vi "Teleop.vi"(10 "Match Info":T1={"Autonomous Elapsed Seconds"=0.0, "TeleOp Elapsed Seconds"=72.473, "Disabled Elapsed Seconds"=26.679, "Visited Autonomous"=FALSE, "Visited TeleOp"=TRUE, "Visited Disabled"=TRUE, "Autonomous Settings"={"Autonomous Style"=enum."Independent", "VI Refnum"=refnum}}, 11 "Call Context":T2=enum."Stop") -> ()   [LabVIEW 2014]
doc: "This VI is called for each TeleOp packet received from the DS where the robot is not disabled. It is often used to read from the joysticks and update I/O or to update setpoints for timed control loops. It should complete and return within 20 milliseconds or it may miss DS packets."
uses:
  Robot Global Data.vi
  <vilib>/Rock Robotics/WPI/SafetyOutput/WPI_SafetyOutputConfigMenu.ctl
  <vilib>/Rock Robotics/WPI/Solenoid/Deprecated/WPI_SolenoidSetBool.vi
  <vilib>/Rock Robotics/WPI/DriverStation/WPI_DriverStationMatch Info.ctl
  <vilib>/Rock Robotics/WPI/DriverStation/WPI_DriverStationDerivedRobotMode.ctl
panel:
  in  "Feed_Forwards_Speed":dbl=0.75 step=0.05
  in  "Feed_Backwards_Speed":dbl=-0.5 step=0.05
  in  "Override_Feed_Value":dbl=1.0
  in  "Override_Feed_Enable":bool
  in  "Mantis_Arm_Control_Rate":dbl=20.0
  out "Delta_Time":dbl=0.023
  in  "Triger_Fire_Threshold":dbl=0.6 format="%#_13g"
  in  "Mantis_Arms_Full_Forward_Position":dbl=69.0
  in  "Mantis_Arms_Full_Back_Position":dbl=100.0
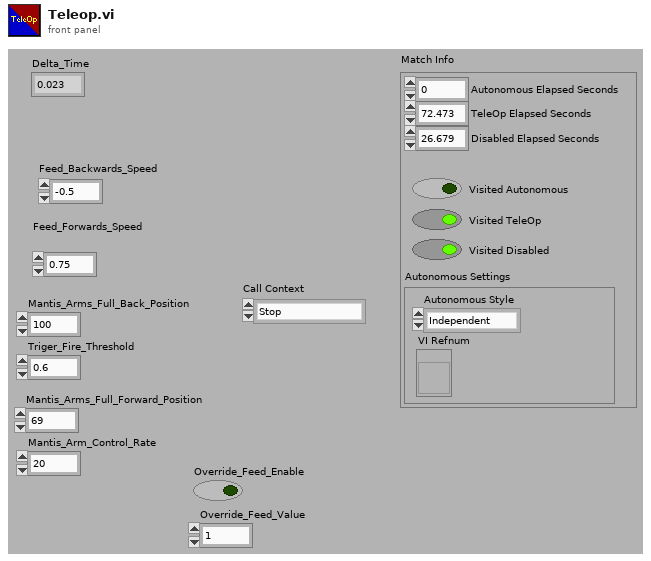
[diagram p1: front panel]
types:
  T1 = typedef "WPI_DriverStationMatch Info.ctl" = cluster{"Autonomous Elapsed Seconds":dbl, "TeleOp Elapsed Seconds":dbl, "Disabled Elapsed Seconds":dbl, "Visited Autonomous":bool, "Visited TeleOp":bool, "Visited Disabled":bool, "Autonomous Settings":cluster{"Autonomous Style":enum16{"Iterative", "Independent"}, "VI Refnum":refnum<vi>}}
  T2 = typedef "WPI_DriverStationDerivedRobotMode.ctl" = enum16{"Init", "Execute", "Stop"}
  T3 = typedef "WPI_SafetyOutputConfigMenu.ctl" = enum16{"Enable", "Disable"}
  T4 = typedef "WPI_RobotDriveDevRef.ctl" = cluster{"DevStatus":errorcluster, "Motors[]":T5[], "Square Inputs":bool, "Max Output":dbl}
  T5 = typedef "WPI_MotorControlDeviceRef.ctl" = cluster{"DeviceStatus":errorcluster, "Type":enum16{"PWM", "CAN"}, "PWM":cluster{"Digital Module":T6, "PWM Channel":T7, "DeadBand":T8}, "CAN":cluster{"Device Number":u8, "Control Mode":T9, "Semaphore":T10, "Max Vout":dbl}, "Invert":bool, "TransformRef":T11, "InvTransformRef":T11}
  T6 = typedef "FPGA_TypedefDigitalModule.ctl" = enum16{"Digital Module 1", "Digital Module 2"}
  T7 = typedef "FPGA_DIOPWMChannel.ctl" = enum8{"PWM 1", "PWM 2", "PWM 3", "PWM 4", "PWM 5", "PWM 6", "PWM 7", "PWM 8", "PWM 9", "PWM 10", "Invalid"}
  T8 = typedef "WPI_PWMDeadband.ctl" = cluster{"Name":string, "maxPositivePwm":i32, "minPositivePwm":i32, "centerPwm":i32, "maxNegativePwm":i32, "minNegativePwm":i32, "angularRange":u16}
  T9 = typedef "WPI_CANJaguar_ControlMode.ctl" = enum8{"Percent VBus", "Current", "Speed", "Position", "Voltage"}
  T10 = typedef "Semaphore RefNum" = refnum<k1>
  T11 = typedef "WPI_PWMTransform_ConPane.ctl" = refnum<vi>
  T12 = typedef "WPI_JoystickDevRef.ctl" = cluster{"Device":T13}
  T13 = typedef "WPI_JoystickDeviceEnum.ctl" = enum16{"USB 0", "USB 1", "USB 2", "USB 3", "USB 4", "USB 5"}
  T14 = cluster{"Button 1":bool, "Button 2":bool, "Button 3":bool, "Button 4":bool, "Button 5":bool, "Button 6":bool, "Button 7":bool, "Button 8":bool, "Button 9":bool, "Button 10":bool, "Button 11":bool, "Button 12":bool}
  T15 = cluster{"axis 1 (x)":dbl, "axis 2 (y)":dbl, "axis 3 (throttle)":dbl, "axis 4":dbl, "axis 5":dbl, "axis 6":dbl}
  T16 = typedef "WPI_SolenoidDevRef.ctl" = cluster{"DevStatus":errorcluster, "Solenoid Module":T17, "Forward Solenoid Channel":T18, "Reverse Solenoid Channel":T18}
  T17 = typedef "FPGA_TypedefSolenoidModule.ctl" = enum16{"Solenoid Module 1", "Solenoid Module 2"}
  T18 = typedef "WPI_SolenoidChannel.ctl" = enum8{"Solenoid 1", "Solenoid 2", "Solenoid 3", "Solenoid 4", "Solenoid 5", "Solenoid 6", "Solenoid 7", "Solenoid 8", "Invalid"}
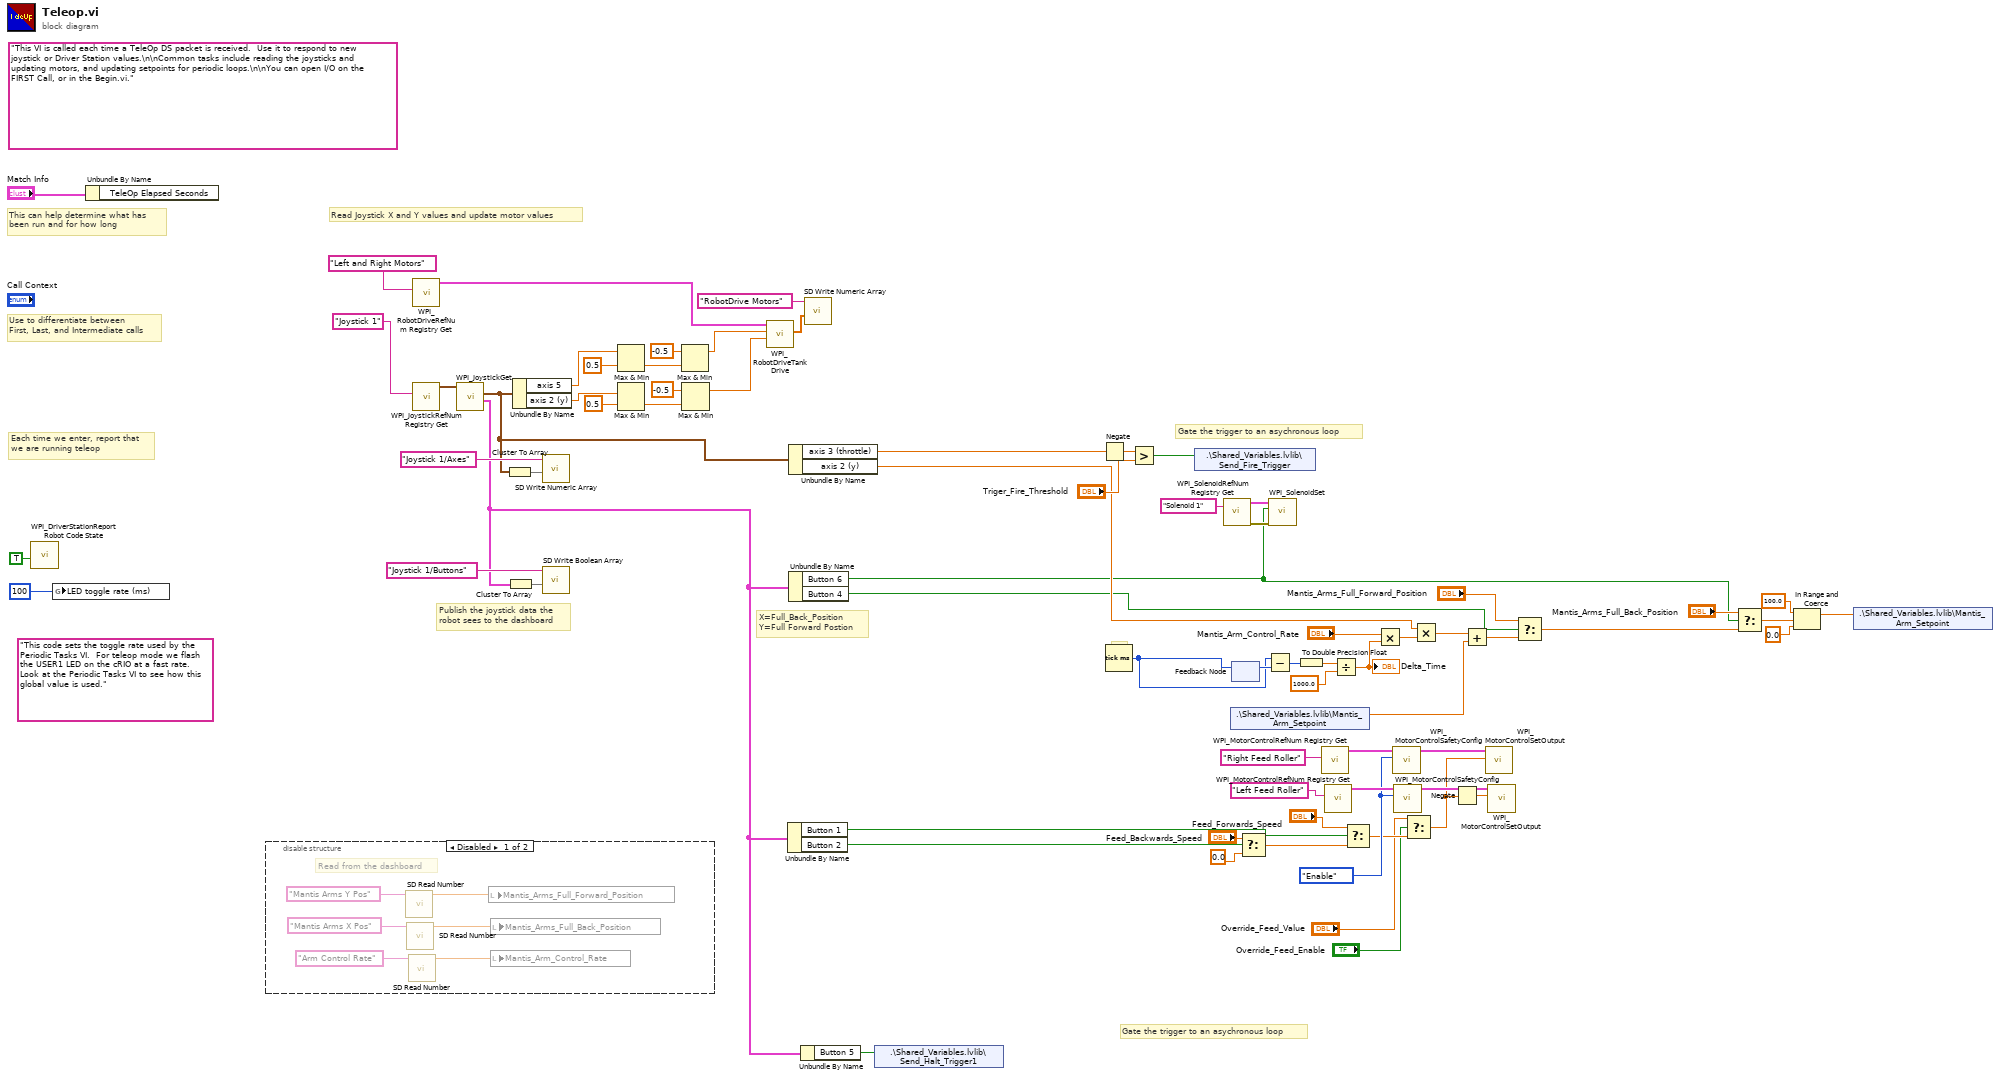
[diagram p0: block diagram]
diagram:
  w31 = WPI_SafetyOutputConfigMenu."Enable" ("mode")
  (unwired) "This code sets the toggle rate used by the Periodic Tasks VI.  For teleop mode we flash the USER1 LED on the cRIO at a fast rate.  Look at the Periodic Tasks VI to see how this global value is used."
  (unwired) "This VI is called each time a TeleOp DS packet is received.  Use it to respond to new joystick or Driver Station values.\n\nCommon tasks include reading the joysticks and updating motors, and updating setpoints for periodic loops.\n\nYou can open I/O on the FIRST Call, or in the Begin.vi."
  # "Gate the trigger to an asychronous loop"
  # "Gate the trigger to an asychronous loop"
  # "dT"
  # "X=Full_Back_Position\nY=Full Forward Postion"
  # "Publish the joystick data the\nrobot sees to the dashboard"
  # "Each time we enter, report that\nwe are running teleop"
  # "Use to differentiate between\nFirst, Last, and Intermediate calls"
  # "This can help determine what has\nbeen run and for how long"
  # "Read Joystick X and Y values and update motor values"
  n1 = call <vilib>:"WPI_DriverStationReport Robot Code State.vi"("TeleOp"=TRUE ("Autonomous")) -> ()  [unwired: 10 in, 1 out]
  n2 = global write "Robot Global Data.vi" "LED toggle rate (ms)"(u32 100 ("LED ms toggle rate")) -> ()
  n3 = Unbundle By Name("Match Info") -> ()  [unwired: 1 out]
  n4 = disable-structure shown="Disabled" {
    frame Disabled {
      # "Read from the dashboard"
      n5 = call <vilib>:"SD Read Number.vi"("Name"="Mantis Arms Y Pos" ("refnum name")) -> ("Numeric"=w74:dbl)  [unwired: 8 in, 2 out]
      n6 = call <vilib>:"SD Read Number.vi"("Name"="Mantis Arms X Pos" ("refnum name")) -> ("Numeric"=w76:dbl)  [unwired: 8 in, 2 out]
      n7 = call <vilib>:"SD Read Number.vi"("Name"="Arm Control Rate" ("refnum name")) -> ("Numeric"=w77:dbl)  [unwired: 8 in, 2 out]
      n8 = local write "Mantis_Arms_Full_Forward_Position"(w74) -> ()
      n9 = local write "Mantis_Arms_Full_Back_Position"(w76) -> ()
      n10 = local write "Mantis_Arm_Control_Rate"(w77) -> ()
    }
    frame Enabled {
    }
  }
  n11 = call <vilib>:"WPI_RobotDriveRefNum Registry Get.vi"("refnum name"="Left and Right Motors") -> ("RobotDriveDevRef"=w62:T4)  [unwired: 1 in, 9 out]
  n12 = call <vilib>:"WPI_JoystickRefNum Registry Get.vi"("refnum name"="Joystick 1") -> ("JoystickDevRef"=w69:T12)  [unwired: 1 in, 9 out]
  n13 = call <vilib>:"WPI_JoystickGet.vi"("JoystickDevRef"=w69) -> ("Buttons"=w12:T14, "Axes"=w11:T15)  [unwired: 1 in, 4 out]
  n14 = Cluster To Array(cluster=w11) -> (array=w64:dbl[])
  n15 = Cluster To Array(cluster=w12) -> (array=w66:bool[])
  n16 = Unbundle By Name(w11) -> ("axis 5"=w10:dbl, "axis 2 (y)"=w9:dbl)
  n17 = call <vilib>:"SD Write Numeric Array.vi"("Numeric Array"=w64, "Name"="Joystick 1/Axes") -> ()  [unwired: 8 in, 2 out]
  n18 = call <vilib>:"SD Write Boolean Array.vi"("Boolean Array"=w66, "Name"="Joystick 1/Buttons") -> ()  [unwired: 8 in, 2 out]
  n19 = Max & Min(x=w10, y=0.5) -> (min(x,y)=w6:dbl)  [unwired: 1 out]
  n20 = Max & Min(x=w9, y=0.5) -> (min(x,y)=w5:dbl)  [unwired: 1 out]
  n21 = Max & Min(x=-0.5, y=w6) -> (max(x,y)=w2:dbl)  [unwired: 1 out]
  n22 = Max & Min(x=-0.5, y=w5) -> (max(x,y)=w1:dbl)  [unwired: 1 out]
  n23 = call <vilib>:"WPI_RobotDriveTankDrive.vi"("Right axis value"=w1, "Left axis value"=w2, "RobotDriveDevRef"=w62) -> ("Motor Values"=w60:dbl[])  [unwired: 6 in, 2 out]
  n24 = Unbundle By Name(w12) -> ("Button 1"=w58:bool, "Button 2"=w57:bool)
  n25 = Unbundle By Name(w11) -> ("axis 3 (throttle)"=w55:dbl, "axis 2 (y)"=w43:dbl)
  n26 = Unbundle By Name(w12) -> ("Button 6"=w13:bool, "Button 4"=w14:bool)
  n27 = Unbundle By Name(w12) -> ("Button 5"=w20:bool)
  n28 = call <vilib>:"SD Write Numeric Array.vi"("Numeric Array"=w60, "Name"="RobotDrive Motors") -> ()  [unwired: 8 in, 2 out]
  n29 = shared-variable ".\\Shared_Variables.lvlib\\Send_Halt_Trigger1"(w20) -> ()  [unwired: 1 in, 1 out]
  n30 = Negate(x=w55) -> (-x=w52:dbl)
  n31 = Tick Count (ms)() -> (millisecond timer value=w50:u32)
  n32 = Greater?(x=w52, y="Triger_Fire_Threshold") -> (0:w21:bool)
  n33 = shared-variable ".\\Shared_Variables.lvlib\\Send_Fire_Trigger"(w21) -> ()  [unwired: 1 in, 1 out]
  n34 = call <vilib>:"WPI_SolenoidRefNum Registry Get.vi"("refnum name"="Solenoid 1") -> ("error out"=w17:errorcluster, "SolenoidDevRef"=w16:T16)  [unwired: 9 in]
  n35 = shared-variable ".\\Shared_Variables.lvlib\\Mantis_Arm_Setpoint"() -> (w36:dbl)  [unwired: 1 in, 1 out]
  n36 = feedback-in #1(w50) -> ()
  n37 = feedback #1() -> (w51:u32)  [unwired: 1 in]
  n38 = Select(t="Feed_Backwards_Speed", s=w57, f=0.0) -> (s? t:f=w30:dbl)
  n39 = Subtract(x=w50, y=w51) -> (x-y=w49:u32)
  n40 = call-poly <vilib>:"WPI_SolenoidSet.vi"("error in (no error)"=w17, "Value"=w13, "SolenoidDevRef"=w16) -> ()  [unwired: 7 in, 2 out]
  n41 = To Double Precision Float(number=w49) -> (double precision float=w48:dbl)
  n42 = call <vilib>:"WPI_MotorControlRefNum Registry Get.vi"("refnum name"="Right Feed Roller") -> ("MotorControlDevRef"=w32:T5)  [unwired: 9 in, 1 out]
  n43 = call <vilib>:"WPI_MotorControlRefNum Registry Get.vi"("refnum name"="Left Feed Roller") -> ("MotorControlDevRef"=w35:T5)  [unwired: 9 in, 1 out]
  n44 = Divide(x=w48, y=1000.0) -> (x/y=w46:dbl)
  "Delta_Time" <- w46
  n45 = Select(t="Feed_Forwards_Speed", s=w58, f=w30) -> (s? t:f=w28:dbl)
  n46 = Multiply(x="Mantis_Arm_Control_Rate", y=w46) -> (x*y=w44:dbl)
  n47 = call <vilib>:"WPI_MotorControlSafetyConfig.vi"("mode"=w31, "MotorControlDevRef"=w32) -> ("MotorControlDevRef"=w33:T5)  [unwired: 8 in, 1 out]
  n48 = call <vilib>:"WPI_MotorControlSafetyConfig.vi"("mode"=w31, "MotorControlDevRef"=w35) -> ("MotorControlDevRef"=w34:T5)  [unwired: 8 in, 1 out]
  n49 = Select(t="Override_Feed_Value", s="Override_Feed_Enable", f=w28) -> (s? t:f=w29:dbl)
  n50 = Multiply(x=w43, y=w44) -> (x*y=w42:dbl)
  n51 = Negate(x=w29) -> (-x=w25:dbl)
  n52 = Add(x=w42, y=w36) -> (x+y=w38:dbl)
  n53 = call <vilib>:"WPI_MotorControlSetOutput.vi"("Output"=w29, "MotorControlDevRef"=w33) -> ()  [unwired: 7 in, 3 out]
  n54 = call <vilib>:"WPI_MotorControlSetOutput.vi"("Output"=w25, "MotorControlDevRef"=w34) -> ()  [unwired: 7 in, 3 out]
  n55 = Select(t="Mantis_Arms_Full_Forward_Position", s=w14, f=w38) -> (s? t:f=w39:dbl)
  n56 = Select(t="Mantis_Arms_Full_Back_Position", s=w13, f=w39) -> (s? t:f=w37:dbl)
  n57 = In Range and Coerce(upper limit=100.0, x=w37, lower limit=0.0) -> (coerced(x)=w24:dbl)  [unwired: 1 out]
  n58 = shared-variable ".\\Shared_Variables.lvlib\\Mantis_Arm_Setpoint"(w24) -> ()  [unwired: 1 in, 1 out]
